vi "ProtoBuff - Call Protoc EXE To Decode Message.vi"(8 "error in":errorcluster, 10 "Encoded ProtoBuf Message In":string) -> (0 "error out":errorcluster, 2 "Decoded ProtoBuf Mesage Out":string)   [LabVIEW 2020]
doc: "Call the protoc.EXE file, which decodes the ProtoBuf Message.\nPassing an empty string, or invalid ProtoBuf message will result in an error."
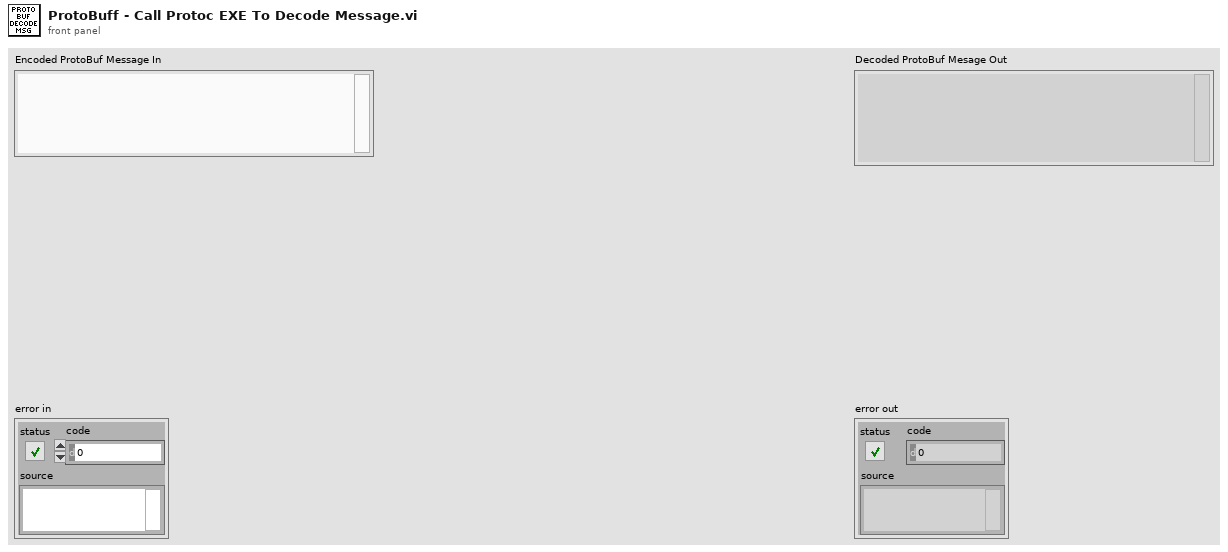
[diagram p1: front panel]
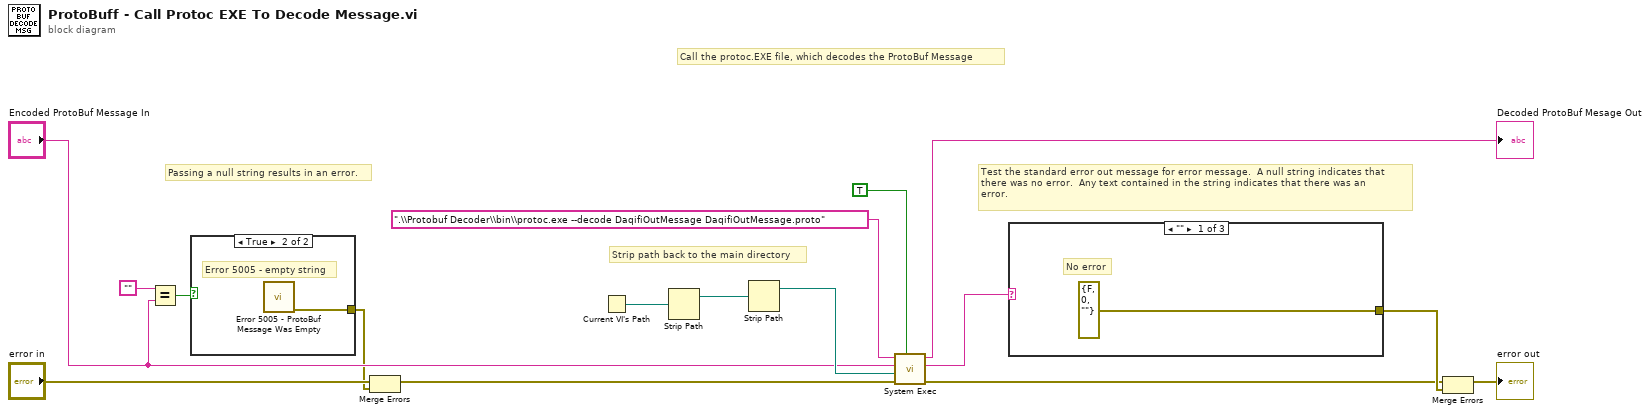
[diagram p0: block diagram]
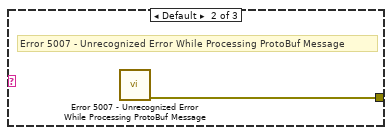
[diagram p2: hidden frame]
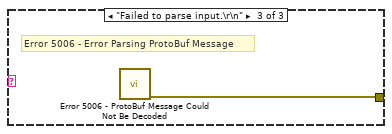
[diagram p3: hidden frame]
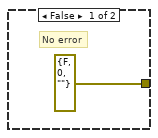
[diagram p4: hidden frame]
diagram:
  # "Passing a null string results in an error."
  # "Test the standard error out message for error message.  A null string indicates that\nthere was no error.  Any text contained in the string indicates that there was an \nerror."
  # "Call the protoc.EXE file, which decodes the ProtoBuf Message"
  # "Strip path back to the main directory"
  n1 = Equal?(x="", y="Encoded ProtoBuf Message In") -> (x = y?=w6:bool)
  n2 = case shown="True" w6 {
    tunnel: [errorcluster {"status"=FALSE, "code"=0, "source"=""} ("error out") w18] -> w5
    frame False {
      # "No error"
    }
    frame True {
      # "Error 5005 - empty string"
      n3 = call "Error 5005 - ProtoBuf Message Was Empty.vi"() -> ("error out"=w18:errorcluster)  [unwired: 11 in]
    }
  }
  n4 = Merge Errors("error in", w5) -> (w7:errorcluster)
  n5 = Current VI's Path() -> (path=w16:path)
  n6 = Strip Path(path=w16) -> (stripped path=w15:path)  [unwired: 1 out]
  n7 = Strip Path(path=w15) -> (stripped path=w14:path)  [unwired: 1 out]
  n8 = call <vilib>:"System Exec.vi"("wait until completion? (T)"=TRUE, "error in (no error)"=w7, "working directory"=w14, "standard input"="Encoded ProtoBuf Message In", "command line"=".\\Protobuf Decoder\\bin\\protoc.exe --decode DaqifiOutMessage DaqifiOutMessage.proto") -> ("error out"=w2:errorcluster, "standard error"=w1:string, "standard output"=→"Decoded ProtoBuf Mesage Out":string)  [unwired: 3 in, 1 out]
  n9 = case shown="\"\"" w1 {
    tunnel: [errorcluster {"status"=FALSE, "code"=0, "source"=""} ("error out") w20 w21] -> w3
    frame "" {
      # "No error"
    }
    frame Default {
      # "Error 5007 - Unrecognized Error While Processing ProtoBuf Message"
      n10 = call "Error 5007 - Unrecognized Error While Processing ProtoBuf Message.vi"() -> ("error out"=w20:errorcluster)  [unwired: 11 in]
    }
    frame "Failed to parse input.\r\n" {
      # "Error 5006 - Error Parsing ProtoBuf Message"
      n11 = call "Error 5006 - ProtoBuf Message Could Not Be Decoded.vi"() -> ("error out"=w21:errorcluster)  [unwired: 11 in]
    }
  }
  n12 = Merge Errors(w2, w3) -> (→"error out":errorcluster)
